vi "Reanimate Target.vi"() -> ()   [LabVIEW 2017, in "Tests.lvlib" / "Toolkit.lvlib"]
uses:
  Toolkit/Toolkit.lvlib
panel:
  in  "Input":bool[](array[boolean])=[FALSE, FALSE, FALSE, TRUE, FALSE, FALSE]
  out "Any?":bool
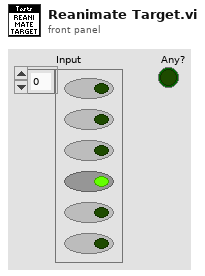
[diagram p1: front panel]
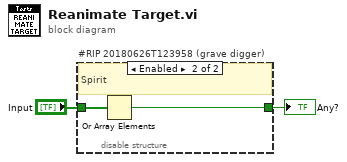
[diagram p0: block diagram]
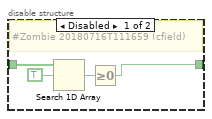
[diagram p2: hidden frame]
diagram:
  n1 = disable-structure "#RIP 20180626T123958 (grave digger)" shown="Enabled" {
    disable-tunnel: "Input" -> [w6 w8]
    disable-tunnel: [w5 w7] -> w1
    frame Disabled {
      # "#Zombie 20180716T111659 (cfield)"
      n2 = Search 1D Array(1D array=w6, element=TRUE) -> (index of element=w3:i32)  [unwired: 1 in]
      n3 = Greater Or Equal To 0?(x=w3) -> (x >= 0?=w5:bool)
    }
    frame Enabled {
      # "Spirit"
      n4 = Or Array Elements(Boolean array=w8) -> (logical OR=w7:bool)
    }
  }
  "Any?" <- w1
